vi "Rotate Robot Points.vi"(4 "ofst":cluster{"left":i32, "top":i32}={"left"=100, "top"=100}, 6 "scale":i32=20, 7 "rotation matrix":T1, 11 "Array in":cluster{"left":dbl, "top":dbl}[](array[cluster])) -> (3 "Array out":cluster{dbl, dbl}[](array[cluster]))   [LabVIEW 2025]
uses:
  <vilib>/Analysis/Matrix/Datatypes/RealMatrix.ctl
  <vilib>/Analysis/baseanly.llb/Vector x A.vi
  <vilib>/Analysis/NI_AALBase.lvlib
  <vilib>/Analysis/Matrix/NI_Matrix.lvlib
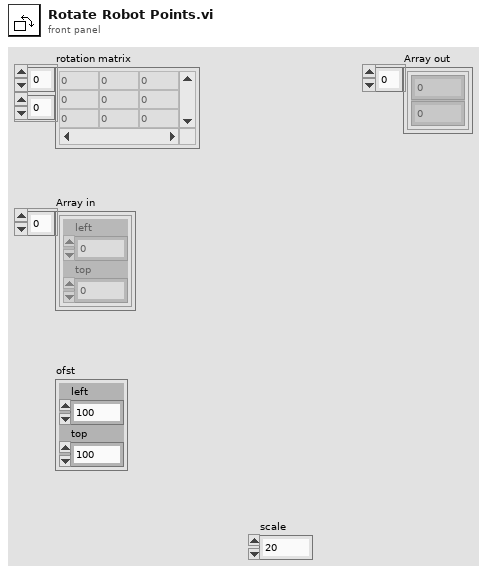
[diagram p1: front panel]
types:
  T1 = typedef "NI_Matrix.lvlib/RealMatrix.ctl" = dbl[][]
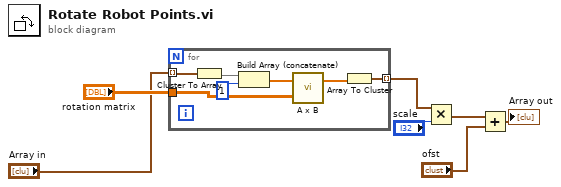
[diagram p0: block diagram]
diagram:
  n1 = for {
    tunnel: "rotation matrix" -> [w14]
    tunnel: "Array in" -> [w13] mode=indexing
    tunnel: [w11] -> w6 mode=indexing
    n2 = Cluster To Array(cluster=w13) -> (array=w10:dbl[])
    n3 = Build Array (concatenate)(w10, 1 ("left")) -> (w8:dbl[])
    n4 = call-poly <vilib>:"A x B.vi"("Matrix A"=w14, "Vector V'"=w8) -> ("V' x A"=w12:dbl[])  [unwired: 1 out]
    n5 = Array To Cluster(array=w12) -> (cluster=w11:cluster{"V' x A[0]":dbl, "V' x A[1]":dbl})
  }
  n6 = Multiply(x=w6, y="scale") -> (x*y=w4:cluster{"V' x A[0]":dbl, "V' x A[1]":dbl}[])
  n7 = Add(x=w4, y="ofst") -> (x+y=→"Array out":cluster{dbl, dbl}[])
